vi "NI9205_driver.vi"(6 "Method NI9205":T1, 7 "MaximumSampleRate?":bool, 8 "error in (no error)":errorcluster, 9 "Number of Samples":i32=100, 10 "SampleRate":dbl=1000.0 format="%0.2f", 11 "Channels NI9205":tag="cDAQ1Mod3/ai0,cDAQ1Mod3/ai2") -> (0 "error out":errorcluster, 2 "SampClk.MaxRate":dbl, 3 "Waveform Graph":waveform(dbl)[](graph), 5 "task out":refnum<k21>)   [LabVIEW 2020]
uses:
  TYPEDEF/NI9205_TD_Method.ctl
  <vilib>/DAQmx/read.llb/DAQmx Read (Analog 1D Wfm NChan NSamp).vi
  <vilib>/DAQmx/miscellaneous.llb/DAQmx Fill In Error Info.vi
  <resource>/objmgr/daqmx.rc
  <vilib>/Waveform/WDTOps.llb/WDT Get Waveform Time Array DBL.vi
panel:
  out "Init?":bool=TRUE
  out "ArrayDeltaTime(sec)":dbl[](array[numeric])
  out "SampQuant.SampPerChan":dbl
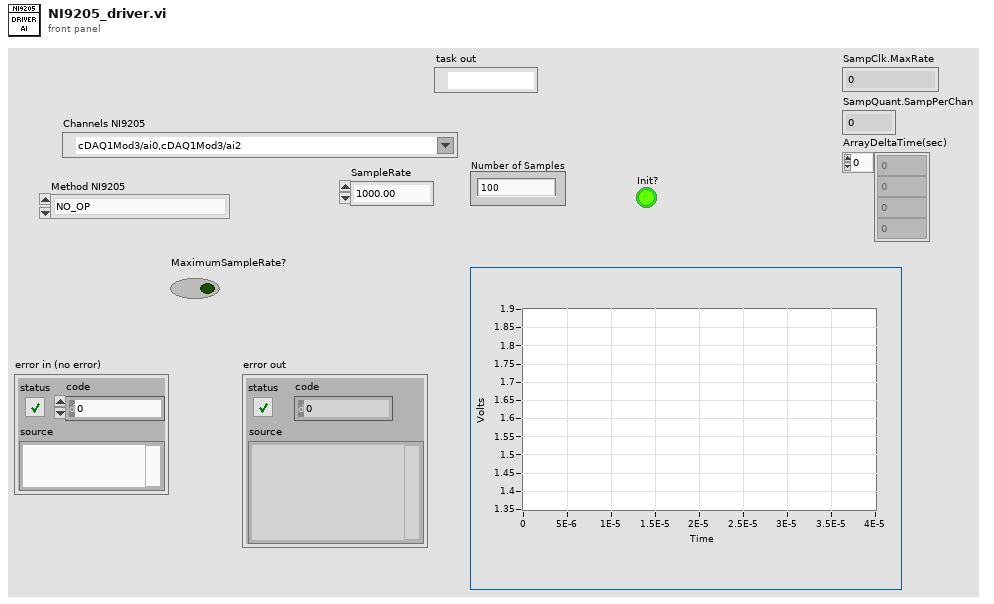
[diagram p1: front panel]
types:
  T1 = typedef "NI9205_TD_Method.ctl" = enum16{"NO_OP", "INIT", "SET", "GET", "CLOSE"}
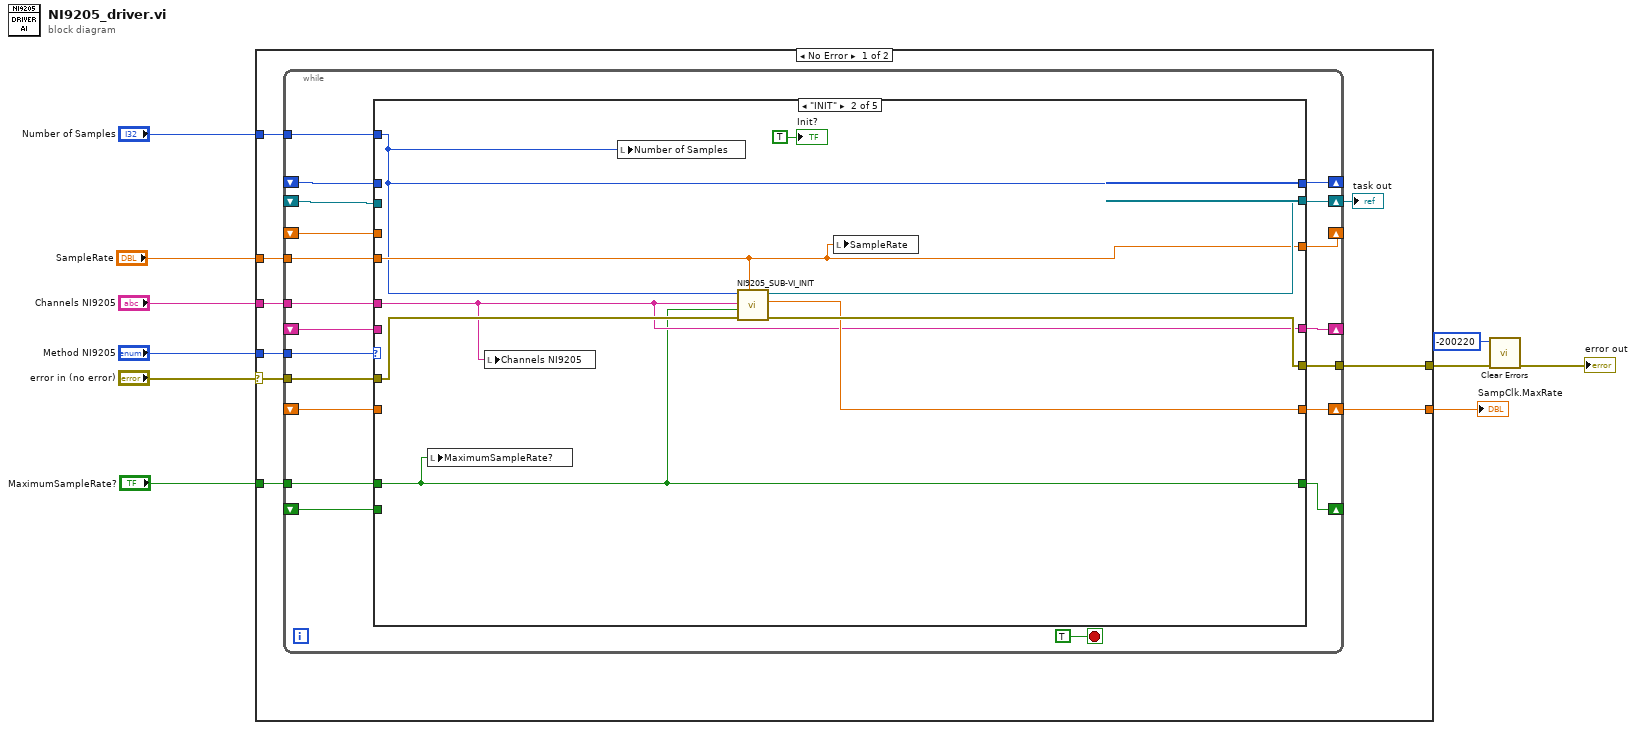
[diagram p0: block diagram]
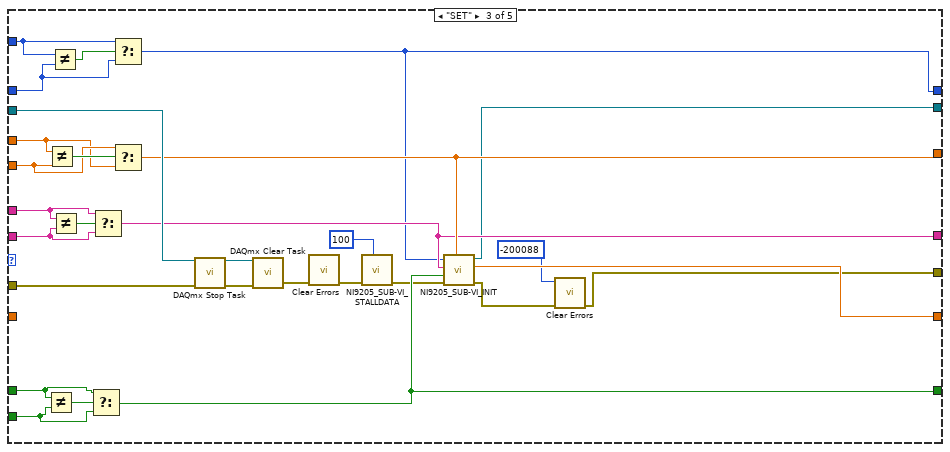
[diagram p3: hidden frame]
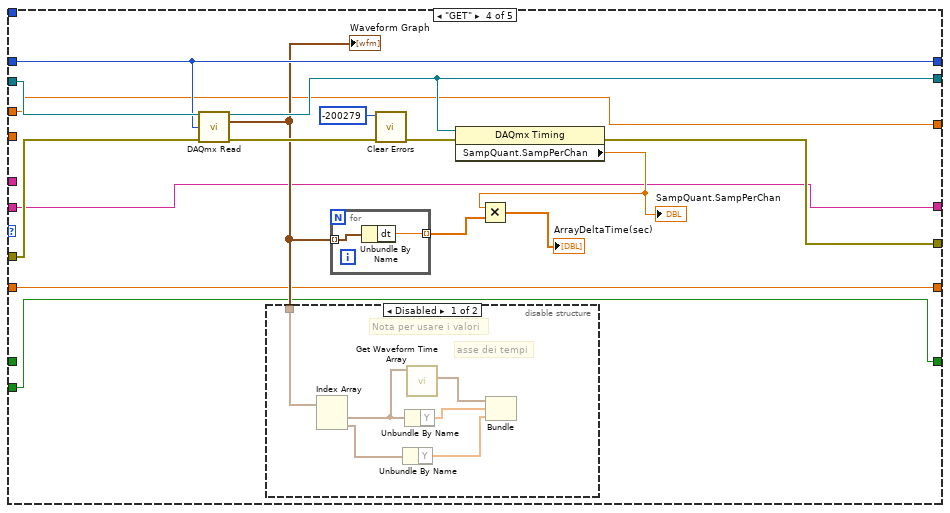
[diagram p4: hidden frame]
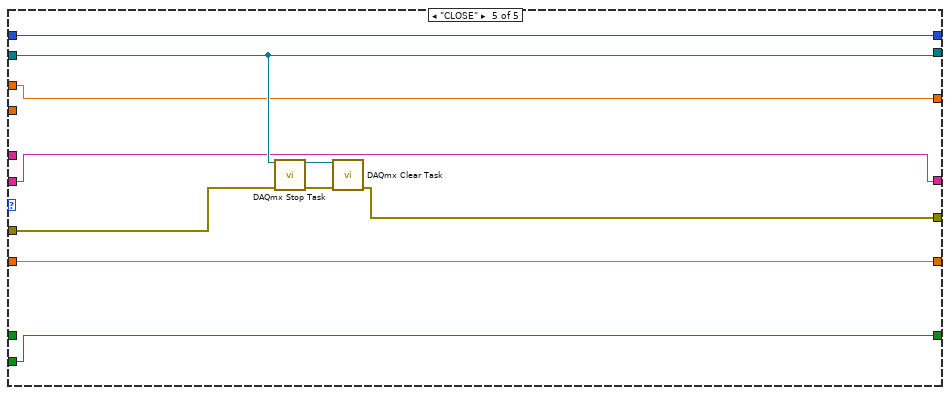
[diagram p6: hidden frame]
diagram:
  n1 = case shown="No Error" "error in (no error)" {
    selector: "error in (no error)" -> [w18 w119]
    tunnel: [w17 w119] -> w9
    tunnel: "Method NI9205" -> [w19 _]
    tunnel: "Channels NI9205" -> [w16 _]
    tunnel: [w15 _] -> w6
    tunnel: "Number of Samples" -> [w14 _]
    tunnel: "SampleRate" -> [w13 _]
    tunnel: "MaximumSampleRate?" -> [w12 _]
    frame No Error {
      n2 = while {
        tunnel: w19 -> [w38]
        shift-right: [w37] -> w11
        shift-left: _ -> [w33]
        shift-right: [w36] -> _
        shift-left: _ -> [w35]
        tunnel: w16 -> [w31]
        tunnel: w18 -> [w34]
        tunnel: [w32] -> w17
        shift-right: [w30] -> w15
        shift-left: _ -> [w29]
        tunnel: w14 -> [w28]
        tunnel: w13 -> [w27]
        tunnel: w12 -> [w26]
        shift-right: [w25] -> _
        shift-left: _ -> [w24]
        shift-right: [w23] -> _
        shift-left: _ -> [w22]
        shift-right: [w21] -> _
        shift-left: _ -> [w20]
        stop <- TRUE stop-if-true
        n3 = case shown="\"INIT\"" w38 {
          tunnel: [w45 w53 w64 w97 w113] -> w37
          tunnel: [w46 w50 w65 w99 w118] -> w36
          tunnel: w35 -> [w46 _ w71 w99 w118]
          tunnel: w34 -> [w44 w55 w82 w98 w115]
          tunnel: w33 -> [w45 _ w80 w100 w113]
          tunnel: [w44 w54 w56 w96 w114] -> w32
          tunnel: w31 -> [_ w49 w78 _ _]
          tunnel: [w43 w52 w63 w91 w112] -> w30
          tunnel: w29 -> [w43 _ _ w91 w112]
          tunnel: w28 -> [_ w50 w72 _ _]
          tunnel: w27 -> [_ w51 w75 _ _]
          tunnel: w26 -> [_ w48 w69 _ _]
          tunnel: [w40 w51 w67 w85 w109] -> w25
          tunnel: w24 -> [w40 _ w74 w85 w109]
          tunnel: [w42 w49 w66 w87 w111] -> w23
          tunnel: w22 -> [w42 _ w77 w87 w111]
          tunnel: [w41 w48 w62 w86 w110] -> w21
          tunnel: w20 -> [w41 _ w68 w86 w110]
          frame "NO_OP", Default {
          }
          frame "INIT" {
            n4 = local write "MaximumSampleRate?"(w48) -> ()
            n5 = local write "Channels NI9205"(w49) -> ()
            n6 = local write "Number of Samples"(w50) -> ()
            n7 = call "NI9205_SUB-VI_INIT.vi"("SampleRate"=w51, "error in (no error)"=w55, "MaximumSampleRate?"=w48, "Channels NI9205"=w49, "Number of Samples"=w50) -> ("error out"=w54:errorcluster, "SampClk.MaxRate"=w52:dbl, "Refnum out"=w53:refnum<k21>)  [unwired: 3 in, 1 out]
            n8 = local write "SampleRate"(w51) -> ()
            "Init?" <- TRUE ("Boolean")
          }
          frame "SET" {
            n9 = Not Equal?(x=w69, y=w68) -> (x != y?=w70:bool)
            n10 = Not Equal?(x=w74, y=w75) -> (x != y?=w76:bool)
            n11 = Not Equal?(x=w72, y=w71) -> (x != y?=w73:bool)
            n12 = Not Equal?(x=w78, y=w77) -> (x != y?=w79:bool)
            n13 = Select(t=w69, s=w70, f=w68) -> (s? t:f=w62:bool)
            n14 = Select(t=w78, s=w79, f=w77) -> (s? t:f=w66:tag)
            n15 = Select(t=w72, s=w73, f=w71) -> (s? t:f=w65:i32)
            n16 = Select(t=w75, s=w76, f=w74) -> (s? t:f=w67:dbl)
            n17 = call <vilib>:"DAQmx Stop Task.vi"("task/channels in"=w80, "error in"=w82) -> ("task out"=w83:refnum<k21>, "error out"=w84:errorcluster)  [unwired: 12 in]
            n18 = call <vilib>:"DAQmx Clear Task.vi"("task in"=w83, "error in"=w84) -> ("error out"=w81:errorcluster)  [unwired: 13 in]
            n19 = call <vilib>:"Clear Errors.vi"("error in (no error)"=w81) -> ("error out"=w61:errorcluster)  [unwired: 5 in, 1 out]
            n20 = call "NI9205_SUB-VI_STALLDATA.vi"("milliseconds to wait"=u32 100, "error in (no error)"=w61) -> ("error out"=w60:errorcluster)  [unwired: 9 in]
            n21 = call "NI9205_SUB-VI_INIT.vi"("SampleRate"=w67, "error in (no error)"=w60, "MaximumSampleRate?"=w62, "Channels NI9205"=w66, "Number of Samples"=w65) -> ("error out"=w57:errorcluster, "SampClk.MaxRate"=w63:dbl, "Refnum out"=w64:refnum<k21>)  [unwired: 3 in, 1 out]
            n22 = call <vilib>:"Clear Errors.vi"("error in (no error)"=w57, "specific error code to clear (0: all)"=-200088) -> ("error out"=w56:errorcluster)  [unwired: 4 in, 1 out]
          }
          frame "GET" {
            n23 = call-poly <vilib>:"DAQmx Read.vi"("task/channels in"=w100, "number of samples per channel"=w99, "error in"=w98) -> ("task out"=w97:refnum<k21>, "data"=w92:waveform(dbl)[], "error out"=w95:errorcluster)  [unwired: 10 in]
            "Waveform Graph" <- w92
            n24 = disable-structure shown="Disabled" {
              disable-tunnel: w92 -> [w104 _]
              frame Disabled {
                # "asse dei tempi"
                # "Nota per usare i valori"
                n25 = Index Array(array=w104) -> (element #1=w103:waveform(dbl), element #2=w106:waveform(dbl))  [unwired: 2 in]
                n26 = Unbundle By Name(w106) -> ("Y"=w105:dbl[])
                n27 = Unbundle By Name(w103) -> ("Y"=w107:dbl[])
                n28 = call-poly <vilib>:"Get Waveform Time Array.vi"("waveform in"=w103) -> ("X array"=w108:timestamp[])  [unwired: 9 in, 1 out]
                n29 = Bundle("X array"=w108, "Y"=w107, "Y"=w105) -> ()  [unwired: 1 in, 1 out]
              }
              frame Enabled {
              }
            }
            n30 = for {
              tunnel: w92 -> [w102] mode=indexing
              tunnel: [w101] -> w90 mode=indexing
              n31 = Unbundle By Name(w102) -> ("dt"=w101:dbl)
            }
            n32 = call <vilib>:"Clear Errors.vi"("error in (no error)"=w95, "specific error code to clear (0: all)"=-200279) -> ("error out"=w94:errorcluster)  [unwired: 4 in, 1 out]
            n33 = property class="DAQmx Timing"(reference=w97, error in=w94) -> (error out=w96:errorcluster, "SampQuant.SampPerChan"=w89:dbl)  [unwired: 1 out]
            "SampQuant.SampPerChan" <- w89
            n34 = Multiply(x=w89, y=w90) -> (x*y=→"ArrayDeltaTime(sec)":dbl[])
          }
          frame "CLOSE" {
            n35 = call <vilib>:"DAQmx Stop Task.vi"("task/channels in"=w113, "error in"=w115) -> ("task out"=w116:refnum<k21>, "error out"=w117:errorcluster)  [unwired: 12 in]
            n36 = call <vilib>:"DAQmx Clear Task.vi"("task in"=w116, "error in"=w117) -> ("error out"=w114:errorcluster)  [unwired: 13 in]
          }
        }
      }
      "task out" <- w11
    }
    frame Error {
    }
  }
  "SampClk.MaxRate" <- w6
  n37 = call <vilib>:"Clear Errors.vi"("error in (no error)"=w9, "specific error code to clear (0: all)"=-200220) -> ("error out"=→"error out":errorcluster)  [unwired: 4 in, 1 out]
